vi "rpcFormat.vi"(9 "Args":string[](array[string]), 10 "method":string, 11 "Name":string) -> (3 "The RPC string":string)   [LabVIEW 2011, in "mbed_LVLibrary.lvlib" / "mbed.lvclass"]
doc: "This VI is used to create the RPC string from the RPC commands. You will only need to use this VI in your own applications if you are developing a new transport mechanism. To execute RPC commands use the RPC function which handles this for you."
uses:
  mbed.lvclass
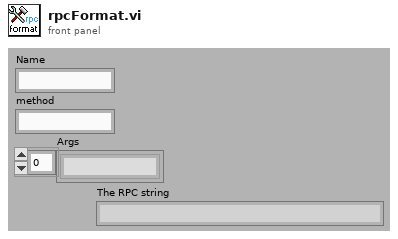
[diagram p1: front panel]
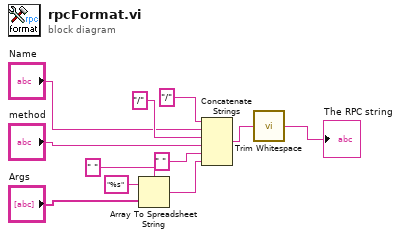
[diagram p0: block diagram]
diagram:
  n1 = Array To Spreadsheet String(delimiter (Tab)=" ", array="Args", 3:"%s" ("format string")) -> (spreadsheet string=w3:string)
  n2 = Concatenate Strings("/" ("string"), "Name", "/" ("string"), "method", " " ("string"), w3) -> (w2:string)
  n3 = call <vilib>:"Trim Whitespace.vi"("string"=w2) -> ("trimmed string"=→"The RPC string":string)  [unwired: 1 in]
